vi "Test.vi"   [LabVIEW 2018]
doc: "This VI is called when test mode begins, and will automatically be terminated when it ends. You can add manual or automatic tests and invoke them from the dashboard."
uses:
  SubSystems/Drive Train/Drive Train Global.vi
  SubSystems/Lift/Lift Global.vi
  SubSystems/Cargo Intake/Cargo Intake Global.vi
  SubSystems/Hatch Panel Intake/Hatch Panel Intake Global.vi
types:
  T1 = enum16{"Manual", "Hatch Panel Zone 1", "Hatch Panel Zone 2", "Hatch Panel Zone 3", "Cargo Zone 1", "Cargo Zone 2", "Cargo Zone 3", "Cargo Ship Zone"}
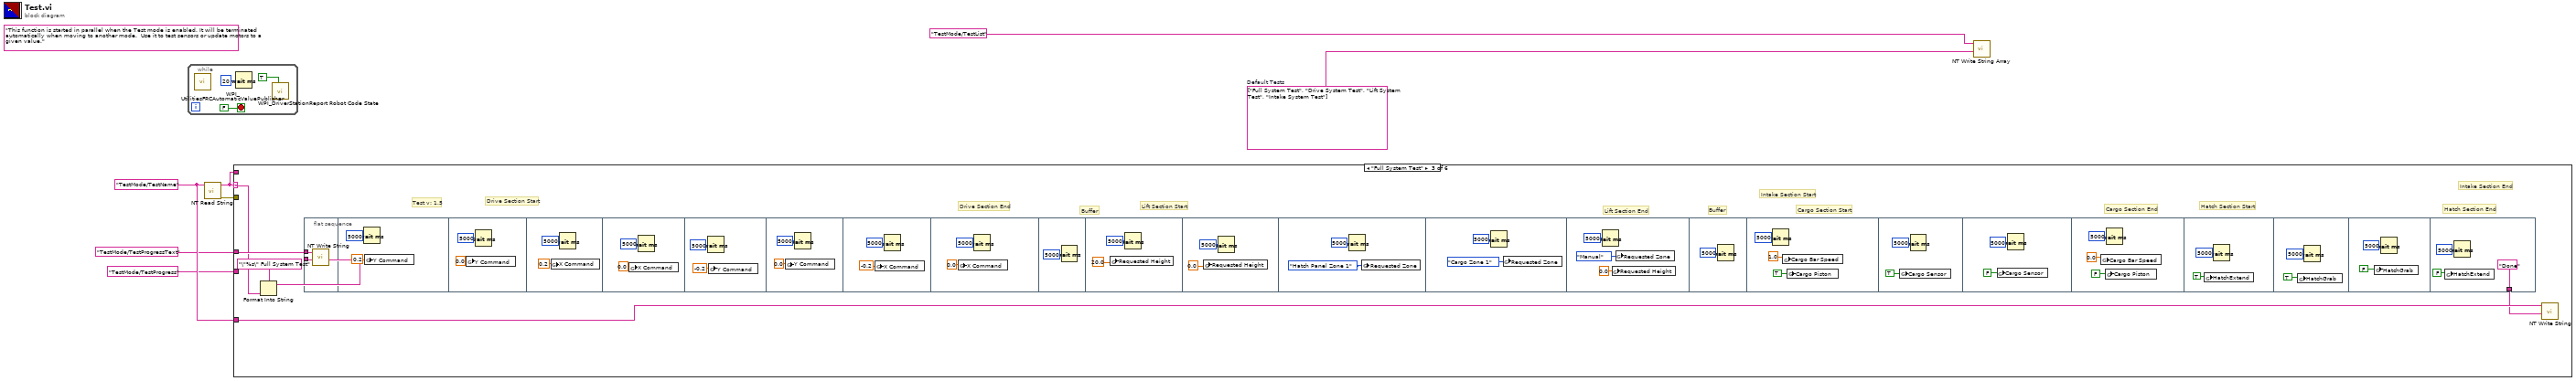
[diagram p0: block diagram]
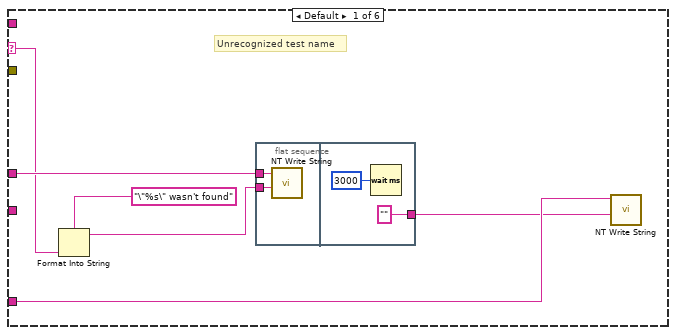
[diagram p2: hidden frame]
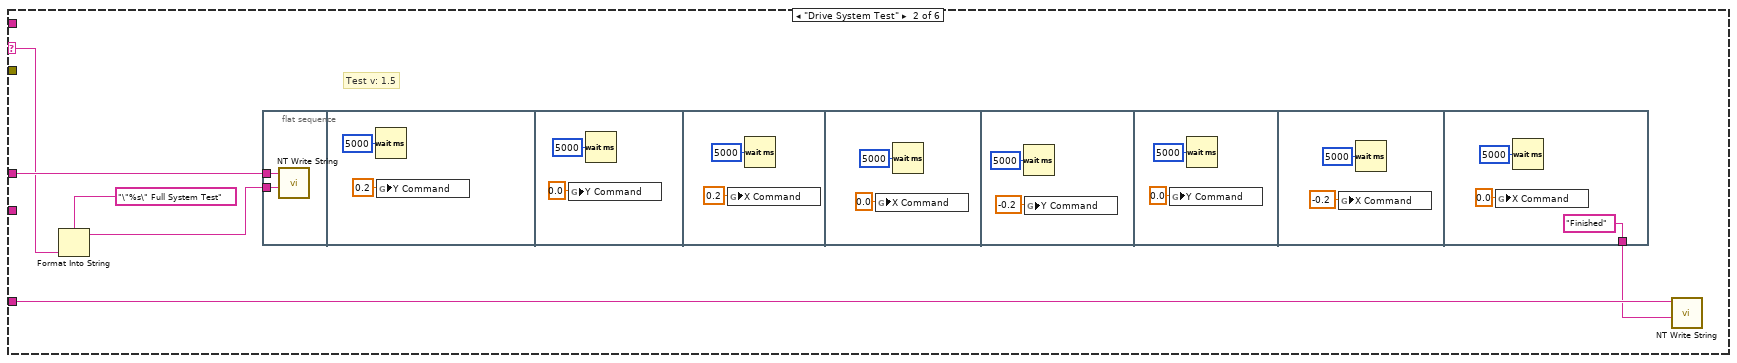
[diagram p3: hidden frame]
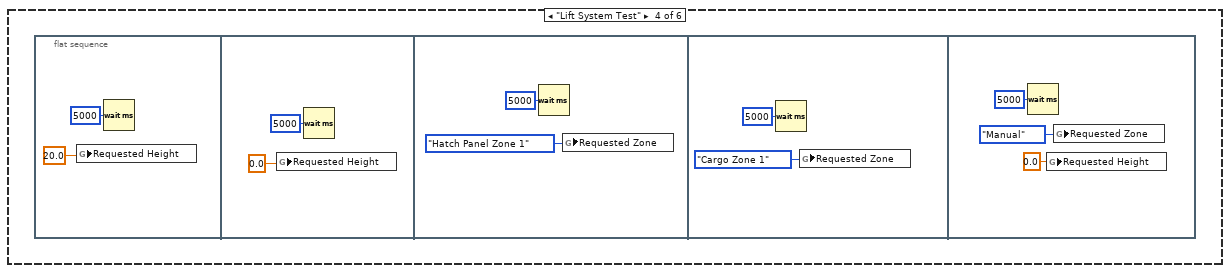
[diagram p4: hidden frame]
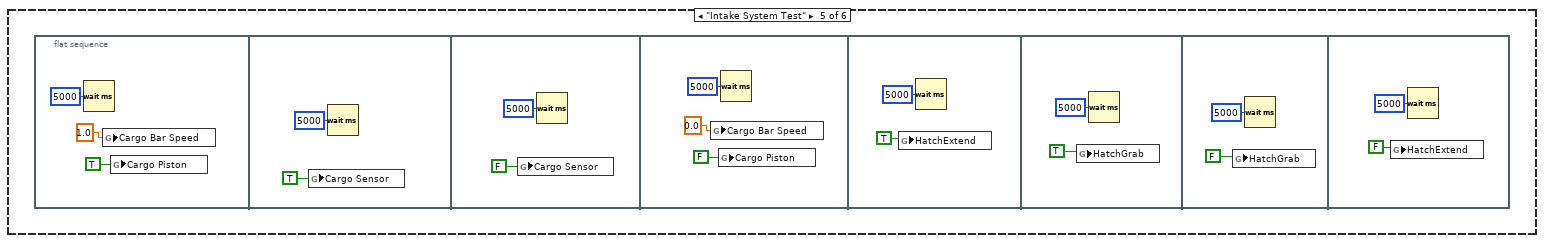
[diagram p5: hidden frame]
diagram:
  w4 = string[] ["Full System Test", "Drive System Test", "Lift System Test", "Intake System Test"]  # Default Tests
  w7 = "TestMode/TestName" ("Name")
  (unwired) "This function is started in parallel when the Test mode is enabled. It will be terminated automatically when moving to another mode.  Use it to test sensors or update motors to a given value."
  n1 = while {
    stop <- FALSE stop-if-true
    n2 = call <vilib>:"WPI_UtilitiesFRCAutomaticValuePublisher.vi"() -> ()  [unwired: 12 in]
    n3 = Wait (ms)(milliseconds to wait=u32 20) -> ()  [unwired: 1 out]
    n4 = call <vilib>:"WPI_DriverStationReport Robot Code State.vi"("Test"=TRUE ("Autonomous")) -> ()  [unwired: 10 in, 1 out]
  }
  n5 = call <vilib>:"NT Read String.vi"("Name"=w7) -> ("error out"=w1:errorcluster, "String"=w2:string)  [unwired: 9 in]
  n6 = case shown="\"Full System Test\"" w2 {
    selector: w2 -> [w15 w25 w50 _ _ _]
    tunnel: w7 -> [w12 w22 w47 _ _ _]
    tunnel: "TestMode/TestProgressText" ("Name") -> [w16 w26 w51 _ _ _]
    tunnel: "TestMode/TestProgress" ("Name") -> [_ _ _ _ _ _]
    tunnel: w2 -> [_ _ _ _ _ _]
    tunnel: w1 -> [_ _ _ _ _ _]
    frame Default {
      # "Unrecognized test name"
      n7 = Format Into String(format string="\"%s\" wasn't found" ("Name"), w15) -> (resulting string=w14:string)  [unwired: 2 in, 1 out]
      n8 = flat-sequence {
        tunnel: w16 -> [w17]
        tunnel: w14 -> [w18]
        tunnel: ["" ("Name")] -> w11
        frame #0 {
          n9 = call <vilib>:"NT Write String.vi"("String"=w18, "Name"=w17) -> ()  [unwired: 9 in, 1 out]
        }
        frame #1 {
          n10 = Wait (ms)(milliseconds to wait=u32 3000) -> ()  [unwired: 1 out]
        }
      }
      n11 = call <vilib>:"NT Write String.vi"("String"=w11, "Name"=w12) -> ()  [unwired: 9 in, 1 out]
    }
    frame "Drive System Test" {
      # "Test v: 1.5"
      n12 = Format Into String(format string="\"%s\" Full System Test" ("Name"), w25) -> (resulting string=w24:string)  [unwired: 2 in, 1 out]
      n13 = flat-sequence {
        tunnel: w26 -> [w27]
        tunnel: w24 -> [w28]
        tunnel: ["Finished"] -> w21
        frame #0 {
          n14 = call <vilib>:"NT Write String.vi"("String"=w28, "Name"=w27) -> ()  [unwired: 9 in, 1 out]
        }
        frame #1 {
          n15 = Wait (ms)(milliseconds to wait=u32 5000) -> ()  [unwired: 1 out]
          n16 = global write "Drive Train Global.vi" "Y Command"(0.2 ("Y Command")) -> ()
        }
        frame #2 {
          n17 = global write "Drive Train Global.vi" "Y Command"(0.0 ("Y Command")) -> ()
          n18 = Wait (ms)(milliseconds to wait=u32 5000) -> ()  [unwired: 1 out]
        }
        frame #3 {
          n19 = global write "Drive Train Global.vi" "X Command"(0.2 ("Y Command")) -> ()
          n20 = Wait (ms)(milliseconds to wait=u32 5000) -> ()  [unwired: 1 out]
        }
        frame #4 {
          n21 = global write "Drive Train Global.vi" "X Command"(0.0 ("Y Command")) -> ()
          n22 = Wait (ms)(milliseconds to wait=u32 5000) -> ()  [unwired: 1 out]
        }
        frame #5 {
          n23 = Wait (ms)(milliseconds to wait=u32 5000) -> ()  [unwired: 1 out]
          n24 = global write "Drive Train Global.vi" "Y Command"(-0.2 ("Y Command")) -> ()
        }
        frame #6 {
          n25 = global write "Drive Train Global.vi" "Y Command"(0.0 ("Y Command")) -> ()
          n26 = Wait (ms)(milliseconds to wait=u32 5000) -> ()  [unwired: 1 out]
        }
        frame #7 {
          n27 = global write "Drive Train Global.vi" "X Command"(-0.2 ("Y Command")) -> ()
          n28 = Wait (ms)(milliseconds to wait=u32 5000) -> ()  [unwired: 1 out]
        }
        frame #8 {
          n29 = global write "Drive Train Global.vi" "X Command"(0.0 ("Y Command")) -> ()
          n30 = Wait (ms)(milliseconds to wait=u32 5000) -> ()  [unwired: 1 out]
        }
      }
      n31 = call <vilib>:"NT Write String.vi"("String"=w21, "Name"=w22) -> ()  [unwired: 9 in, 1 out]
    }
    frame "Full System Test" {
      # "Intake Section End"
      # "Hatch Section End"
      # "Hatch Section Start"
      # "Cargo Section End"
      # "Cargo Section Start"
      # "Intake Section Start"
      # "Buffer"
      # "Lift Section End"
      # "Buffer"
      # "Drive Section End"
      # "Drive Section Start"
      # "Lift Section Start"
      # "Test v: 1.5"
      n32 = Format Into String(format string="\"%s\" Full System Test" ("Name"), w50) -> (resulting string=w49:string)  [unwired: 2 in, 1 out]
      n33 = flat-sequence {
        tunnel: w51 -> [w52]
        tunnel: w49 -> [w53]
        tunnel: ["Done"] -> w46
        frame #0 {
          n34 = call <vilib>:"NT Write String.vi"("String"=w53, "Name"=w52) -> ()  [unwired: 9 in, 1 out]
        }
        frame #1 {
          n35 = Wait (ms)(milliseconds to wait=u32 5000) -> ()  [unwired: 1 out]
          n36 = global write "Drive Train Global.vi" "Y Command"(0.2 ("Y Command")) -> ()
        }
        frame #2 {
          n37 = global write "Drive Train Global.vi" "Y Command"(0.0 ("Y Command")) -> ()
          n38 = Wait (ms)(milliseconds to wait=u32 5000) -> ()  [unwired: 1 out]
        }
        frame #3 {
          n39 = global write "Drive Train Global.vi" "X Command"(0.2 ("Y Command")) -> ()
          n40 = Wait (ms)(milliseconds to wait=u32 5000) -> ()  [unwired: 1 out]
        }
        frame #4 {
          n41 = global write "Drive Train Global.vi" "X Command"(0.0 ("Y Command")) -> ()
          n42 = Wait (ms)(milliseconds to wait=u32 5000) -> ()  [unwired: 1 out]
        }
        frame #5 {
          n43 = Wait (ms)(milliseconds to wait=u32 5000) -> ()  [unwired: 1 out]
          n44 = global write "Drive Train Global.vi" "Y Command"(-0.2 ("Y Command")) -> ()
        }
        frame #6 {
          n45 = global write "Drive Train Global.vi" "Y Command"(0.0 ("Y Command")) -> ()
          n46 = Wait (ms)(milliseconds to wait=u32 5000) -> ()  [unwired: 1 out]
        }
        frame #7 {
          n47 = global write "Drive Train Global.vi" "X Command"(-0.2 ("Y Command")) -> ()
          n48 = Wait (ms)(milliseconds to wait=u32 5000) -> ()  [unwired: 1 out]
        }
        frame #8 {
          n49 = global write "Drive Train Global.vi" "X Command"(0.0 ("Y Command")) -> ()
          n50 = Wait (ms)(milliseconds to wait=u32 5000) -> ()  [unwired: 1 out]
        }
        frame #9 {
          n51 = Wait (ms)(milliseconds to wait=u32 5000) -> ()  [unwired: 1 out]
        }
        frame #10 {
          n52 = global write "Lift Global.vi" "Requested Height"(20.0 ("Requested Height")) -> ()
          n53 = Wait (ms)(milliseconds to wait=u32 5000) -> ()  [unwired: 1 out]
        }
        frame #11 {
          n54 = global write "Lift Global.vi" "Requested Height"(0.0 ("Requested Height")) -> ()
          n55 = Wait (ms)(milliseconds to wait=u32 5000) -> ()  [unwired: 1 out]
        }
        frame #12 {
          n56 = Wait (ms)(milliseconds to wait=u32 5000) -> ()  [unwired: 1 out]
          n57 = global write "Lift Global.vi" "Requested Zone"(T1."Hatch Panel Zone 1" ("Requested Zone")) -> ()
        }
        frame #13 {
          n58 = Wait (ms)(milliseconds to wait=u32 5000) -> ()  [unwired: 1 out]
          n59 = global write "Lift Global.vi" "Requested Zone"(T1."Cargo Zone 1" ("Requested Zone")) -> ()
        }
        frame #14 {
          n60 = Wait (ms)(milliseconds to wait=u32 5000) -> ()  [unwired: 1 out]
          n61 = global write "Lift Global.vi" "Requested Height"(0.0 ("Requested Height")) -> ()
          n62 = global write "Lift Global.vi" "Requested Zone"(T1."Manual" ("Requested Zone")) -> ()
        }
        frame #15 {
          n63 = Wait (ms)(milliseconds to wait=u32 5000) -> ()  [unwired: 1 out]
        }
        frame #16 {
          n64 = Wait (ms)(milliseconds to wait=u32 5000) -> ()  [unwired: 1 out]
          n65 = global write "Cargo Intake Global.vi" "Cargo Bar Speed"(1.0 ("Cargo Bar Speed")) -> ()
          n66 = global write "Cargo Intake Global.vi" "Cargo Piston"(TRUE) -> ()
        }
        frame #17 {
          n67 = global write "Cargo Intake Global.vi" "Cargo Sensor"(TRUE) -> ()
          n68 = Wait (ms)(milliseconds to wait=u32 5000) -> ()  [unwired: 1 out]
        }
        frame #18 {
          n69 = global write "Cargo Intake Global.vi" "Cargo Sensor"(FALSE) -> ()
          n70 = Wait (ms)(milliseconds to wait=u32 5000) -> ()  [unwired: 1 out]
        }
        frame #19 {
          n71 = global write "Cargo Intake Global.vi" "Cargo Bar Speed"(0.0 ("Cargo Bar Speed")) -> ()
          n72 = global write "Cargo Intake Global.vi" "Cargo Piston"(FALSE) -> ()
          n73 = Wait (ms)(milliseconds to wait=u32 5000) -> ()  [unwired: 1 out]
        }
        frame #20 {
          n74 = global write "Hatch Panel Intake Global.vi" "HatchExtend"(TRUE) -> ()
          n75 = Wait (ms)(milliseconds to wait=u32 5000) -> ()  [unwired: 1 out]
        }
        frame #21 {
          n76 = global write "Hatch Panel Intake Global.vi" "HatchGrab"(TRUE) -> ()
          n77 = Wait (ms)(milliseconds to wait=u32 5000) -> ()  [unwired: 1 out]
        }
        frame #22 {
          n78 = global write "Hatch Panel Intake Global.vi" "HatchGrab"(FALSE) -> ()
          n79 = Wait (ms)(milliseconds to wait=u32 5000) -> ()  [unwired: 1 out]
        }
        frame #23 {
          n80 = global write "Hatch Panel Intake Global.vi" "HatchExtend"(FALSE) -> ()
          n81 = Wait (ms)(milliseconds to wait=u32 5000) -> ()  [unwired: 1 out]
        }
      }
      n82 = call <vilib>:"NT Write String.vi"("String"=w46, "Name"=w47) -> ()  [unwired: 9 in, 1 out]
    }
    frame "Lift System Test" {
      n83 = flat-sequence {
        frame #0 {
          n84 = global write "Lift Global.vi" "Requested Height"(20.0 ("Requested Height")) -> ()
          n85 = Wait (ms)(milliseconds to wait=u32 5000) -> ()  [unwired: 1 out]
        }
        frame #1 {
          n86 = global write "Lift Global.vi" "Requested Height"(0.0 ("Requested Height")) -> ()
          n87 = Wait (ms)(milliseconds to wait=u32 5000) -> ()  [unwired: 1 out]
        }
        frame #2 {
          n88 = Wait (ms)(milliseconds to wait=u32 5000) -> ()  [unwired: 1 out]
          n89 = global write "Lift Global.vi" "Requested Zone"(T1."Hatch Panel Zone 1" ("Requested Zone")) -> ()
        }
        frame #3 {
          n90 = Wait (ms)(milliseconds to wait=u32 5000) -> ()  [unwired: 1 out]
          n91 = global write "Lift Global.vi" "Requested Zone"(T1."Cargo Zone 1" ("Requested Zone")) -> ()
        }
        frame #4 {
          n92 = Wait (ms)(milliseconds to wait=u32 5000) -> ()  [unwired: 1 out]
          n93 = global write "Lift Global.vi" "Requested Height"(0.0 ("Requested Height")) -> ()
          n94 = global write "Lift Global.vi" "Requested Zone"(T1."Manual" ("Requested Zone")) -> ()
        }
      }
    }
    frame "Intake System Test" {
      n95 = flat-sequence {
        frame #0 {
          n96 = Wait (ms)(milliseconds to wait=u32 5000) -> ()  [unwired: 1 out]
          n97 = global write "Cargo Intake Global.vi" "Cargo Bar Speed"(1.0 ("Cargo Bar Speed")) -> ()
          n98 = global write "Cargo Intake Global.vi" "Cargo Piston"(TRUE) -> ()
        }
        frame #1 {
          n99 = global write "Cargo Intake Global.vi" "Cargo Sensor"(TRUE) -> ()
          n100 = Wait (ms)(milliseconds to wait=u32 5000) -> ()  [unwired: 1 out]
        }
        frame #2 {
          n101 = global write "Cargo Intake Global.vi" "Cargo Sensor"(FALSE) -> ()
          n102 = Wait (ms)(milliseconds to wait=u32 5000) -> ()  [unwired: 1 out]
        }
        frame #3 {
          n103 = global write "Cargo Intake Global.vi" "Cargo Bar Speed"(0.0 ("Cargo Bar Speed")) -> ()
          n104 = global write "Cargo Intake Global.vi" "Cargo Piston"(FALSE) -> ()
          n105 = Wait (ms)(milliseconds to wait=u32 5000) -> ()  [unwired: 1 out]
        }
        frame #4 {
          n106 = global write "Hatch Panel Intake Global.vi" "HatchExtend"(TRUE) -> ()
          n107 = Wait (ms)(milliseconds to wait=u32 5000) -> ()  [unwired: 1 out]
        }
        frame #5 {
          n108 = global write "Hatch Panel Intake Global.vi" "HatchGrab"(TRUE) -> ()
          n109 = Wait (ms)(milliseconds to wait=u32 5000) -> ()  [unwired: 1 out]
        }
        frame #6 {
          n110 = global write "Hatch Panel Intake Global.vi" "HatchGrab"(FALSE) -> ()
          n111 = Wait (ms)(milliseconds to wait=u32 5000) -> ()  [unwired: 1 out]
        }
        frame #7 {
          n112 = global write "Hatch Panel Intake Global.vi" "HatchExtend"(FALSE) -> ()
          n113 = Wait (ms)(milliseconds to wait=u32 5000) -> ()  [unwired: 1 out]
        }
      }
    }
    frame "" {
      # "No test to run"
    }
  }
  n114 = call <vilib>:"NT Write String Array.vi"("String Array"=w4, "Name"="TestMode/TestList") -> ()  [unwired: 9 in, 1 out]
